vi "PROG 7 - TAKE INPUT TWO NUMBERS AND DISPLAY THEIR SUM AND DIFFERENCE.vi"() -> ()   [LabVIEW 2012]
panel:
  out "Boolean":bool
  out "X1*Y1":dbl
  out "X1-Y1":dbl
  out "X1+Y1":dbl
  in  "Y1":dbl
  in  "X1":dbl
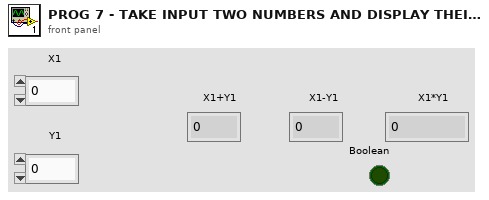
[diagram p1: front panel]
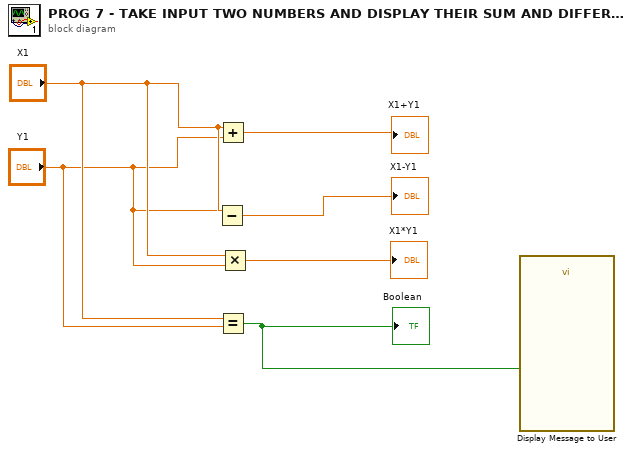
[diagram p0: block diagram]
diagram:
  n1 = Subtract(x="X1", y="Y1") -> (x-y=→"X1-Y1":dbl)
  n2 = Add(x="X1", y="Y1") -> (x+y=→"X1+Y1":dbl)
  n3 = Equal?(x="X1", y="Y1") -> (x = y?=w1:bool)
  "Boolean" <- w1
  n4 = Multiply(x="X1", y="Y1") -> (x*y=→"X1*Y1":dbl)
  n5 = call "Display Message to User"("Enable"=w1) -> ()  [unwired: 9 in, 2 out]
